vi "Initialize.vi"(8 "error out 2":errorcluster) -> (0 "error out":errorcluster, 3 "LV Awesome":refnum<class "LV Awesome.lvclass">)   [LabVIEW 2020, in "LV-Awesome.lvlib" / "LV Awesome.lvclass"]
uses:
  LV Awesome.lvclass
  Data.ctl
  LV Awesome.lvclass/LV Awesome.ctl
  <vilib>/JDP Science/JSONtext/JSONtext.lvlib
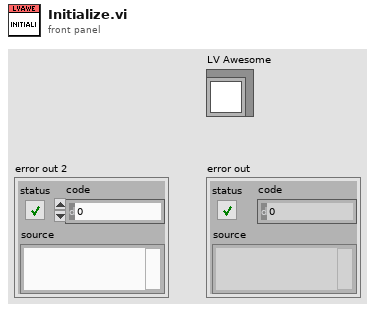
[diagram p1: front panel]
types:
  T1 = typedef "LV-Awesome.lvlib/LV Awesome.lvclass/Data.ctl" = cluster{"Glyphs":map{string, u32}, "Fonts":map{string, path}}
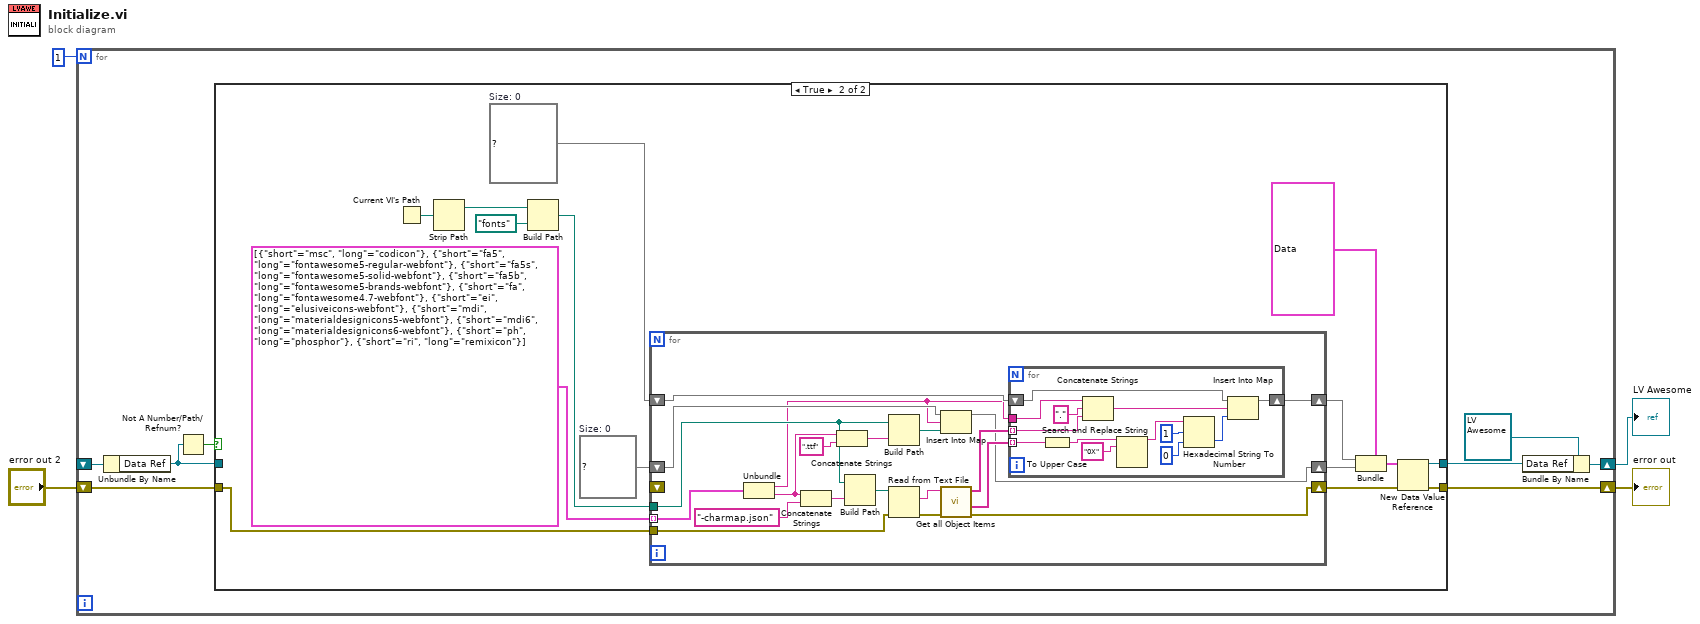
[diagram p0: block diagram]
diagram:
  n1 = for {
    N: 1 -> [_]
    shift-right: [w9] -> w3
    shift-left: _ -> [w10]
    shift-right: [w12] -> w2
    shift-left: "error out 2" -> [w11]
    n2 = Unbundle By Name(w10) -> ("Data Ref"=w6:refnum<data-value>)
    n3 = Not A Number/Path/Refnum?(number/path/refnum=w6) -> (NaN/Path/Refnum?=w8:bool)
    n4 = case shown="True" w8 {
      tunnel: [w14 w15] -> w12
      tunnel: w11 -> [w14 w22]
      tunnel: [w13 w17] -> w7
      tunnel: w6 -> [w13 _]
      frame False {
      }
      frame True {
        w23 = map{string, path} {}  # Size: 0
        w26 = map{string, u32} {}  # Size: 0
        n5 = Current VI's Path() -> (path=w29:path)
        n6 = Strip Path(path=w29) -> (stripped path=w28:path)  [unwired: 1 out]
        n7 = Build Path(base path=w28, name or relative path=path "fonts") -> (appended path=w24:path)
        n8 = for {
          shift-right: [w45] -> w19
          shift-left: w26 -> [w48]
          tunnel: cluster{"short":string, "long":string}[] [{"short"="msc", "long"="codicon"}, {"short"="fa5", "long"="fontawesome5-regular-webfont"}, {"short"="fa5s", "long"="fontawesome5-solid-webfont"}, {"short"="fa5b", "long"="fontawesome5-brands-webfont"}, {"short"="fa", "long"="fontawesome4.7-webfont"}, {"short"="ei", "long"="elusiveicons-webfont"}, {"short"="mdi", "long"="materialdesignicons5-webfont"}, {"short"="mdi6", "long"="materialdesignicons6-webfont"}, {"short"="ph", "long"="phosphor"}, {"short"="ri", "long"="remixicon"}] -> [w43] mode=indexing
          tunnel: w24 -> [w37]
          shift-right: [w32] -> w18
          shift-left: w23 -> [w35]
          shift-right: [w31] -> w16
          shift-left: _ -> [_]
          tunnel: w22 -> [w30]
          n9 = Unbundle(w43) -> ("short"=w34:string, "long"=w39:string)
          n10 = Concatenate Strings(w39, "-charmap.json" ("substring (\"\")")) -> (w41:string)
          n11 = Concatenate Strings(w39, ".ttf" ("string")) -> (w36:string)
          n12 = Build Path(base path=w37, name or relative path=w41) -> (appended path=w40:path)
          n13 = Build Path(base path=w37, name or relative path=w36) -> (appended path=w33:path)
          n14 = Read from Text File(file (use dialog)=w40, error in=w30) -> (text=w49:string, error out=w47:errorcluster)  [unwired: 2 in, 2 out]
          n15 = Insert Into Map(map in=w35, key=w34, value=w33) -> (map out=w32:map{string, path})  [unwired: 2 out]
          n16 = call <vilib>:"Get all Object Items.vi"("error in (no error)"=w47, "JSON"=w49) -> ("error out"=w31:errorcluster, "<JSON>"=w44:string[], "Item Names"=w46:string[])  [unwired: 6 in, 1 out]
          n17 = for {
            shift-right: [w61] -> w45
            shift-left: w48 -> [w62]
            tunnel: w46 -> [w60] mode=indexing
            tunnel: w34 -> [w59]
            tunnel: w44 -> [w57] mode=indexing
            n18 = To Upper Case(1:w57) -> (0:w54:string)
            n19 = Concatenate Strings(w59, "." ("string"), w60) -> (w58:string)
            n20 = Search and Replace String(input string=w54, search string="0X") -> (result string=w52:string)  [unwired: 6 in, 3 out]
            n21 = Hexadecimal String To Number(string=w52, offset=1, default (0uL)=u32 0 ("default (0 U32)")) -> (number=w55:u32)  [unwired: 1 out]
            n22 = Insert Into Map(map in=w62, key=w58, value=w55) -> (map out=w61:map{string, u32})  [unwired: 2 out]
          }
        }
        n23 = Bundle(cluster=T1 {"Glyphs"={}, "Fonts"={}}, "Glyphs"=w19, "Fonts"=w18) -> (w20:T1)
        n24 = New Data Value Reference(data value=w20, error in=w16) -> (data value reference=w17:refnum<data-value>, error out=w15:errorcluster)
      }
    }
    n25 = Bundle By Name(cluster=refnum<class "LV Awesome.lvclass"> refnum ("LV-Awesome.lvlib:LV Awesome.lvclass"), "Data Ref"=w7) -> (w9:refnum<class "LV Awesome.lvclass">)
  }
  "LV Awesome" <- w3
  "error out" <- w2
